vi "Create File.vi"(8 "error in (no error)":errorcluster, 10 "File Name Prefix":string) -> (0 "error out":errorcluster, 3 "refnum out":refnum<file>)   [LabVIEW 2015]
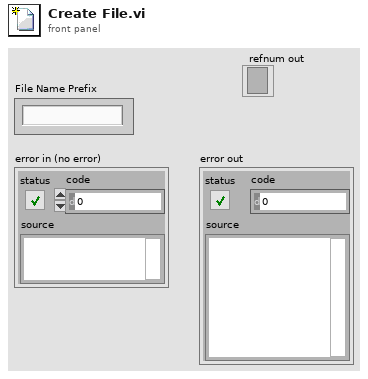
[diagram p1: front panel]
types:
  T1 = enum16{"open", "replace", "create", "open or create", "replace or create", "replace or create with confirmation"}
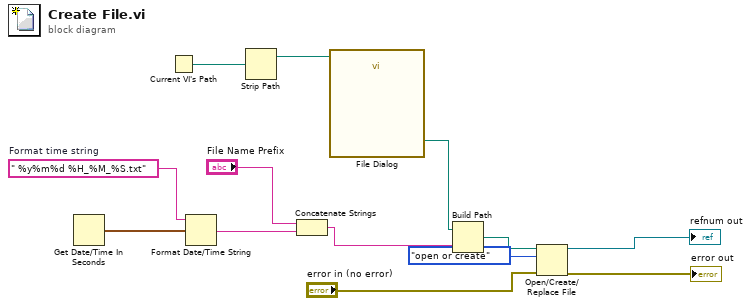
[diagram p0: block diagram]
diagram:
  w12 = " %y%m%d %H_%M_%S.txt"  # Format time string
  n1 = Get Date/Time In Seconds() -> (seconds since 1Jan1904=w10:timestamp)
  n2 = Current VI's Path() -> (path=w4:path)
  n3 = Format Date/Time String(time format string (%c)=w12, seconds (now)=w10) -> (date/time string=w13:string)  [unwired: 1 in]
  n4 = Strip Path(path=w4) -> (stripped path=w3:path)  [unwired: 1 out]
  n5 = Concatenate Strings("File Name Prefix", w13) -> (w9:string)
  n6 = call "File Dialog"("start path"=w3) -> ("selected path"=w8:path)  [unwired: 11 in, 3 out]
  n7 = Build Path(base path=w8, name or relative path=w9) -> (appended path=w7:path)
  n8 = Open/Create/Replace File(file path (use dialog)=w7, error in="error in (no error)", operation (0:open)=T1."open or create") -> (refnum out=→"refnum out":refnum<file>, error out=→"error out":errorcluster)  [unwired: 3 in, 1 out]
